vi "Main.vi"() -> ()   [LabVIEW 2020]
uses:
  Global Variables/Global Number of Indices.vi
  Global Variables/Global Correct Answer.vi
  Global Variables/Global N-Back Setting.vi
  Global Variables/Global User_Answer.vi
  Global Variables/Global Label.vi
  Global Variables/Training_Status.vi
  Global Variables/Number_of_Windows.vi
  Global Variables/Window_Size.vi
  Global Variables/Global Send To ANN.vi
  Global Variables/Trainning Done.vi
  Global Variables/Global Difficulty Level.vi
  Global Variables/Global Enable Logging.vi
  Global Variables/Global_Rating.vi
panel:
  out "Difficulty Level":u8
  out "tiggerTime":u32
  out "New square":T1
  out "seq":i8
  out "Data":bool[](array[boolean])
  out "error out":errorcluster
  out "2D Picture":picture
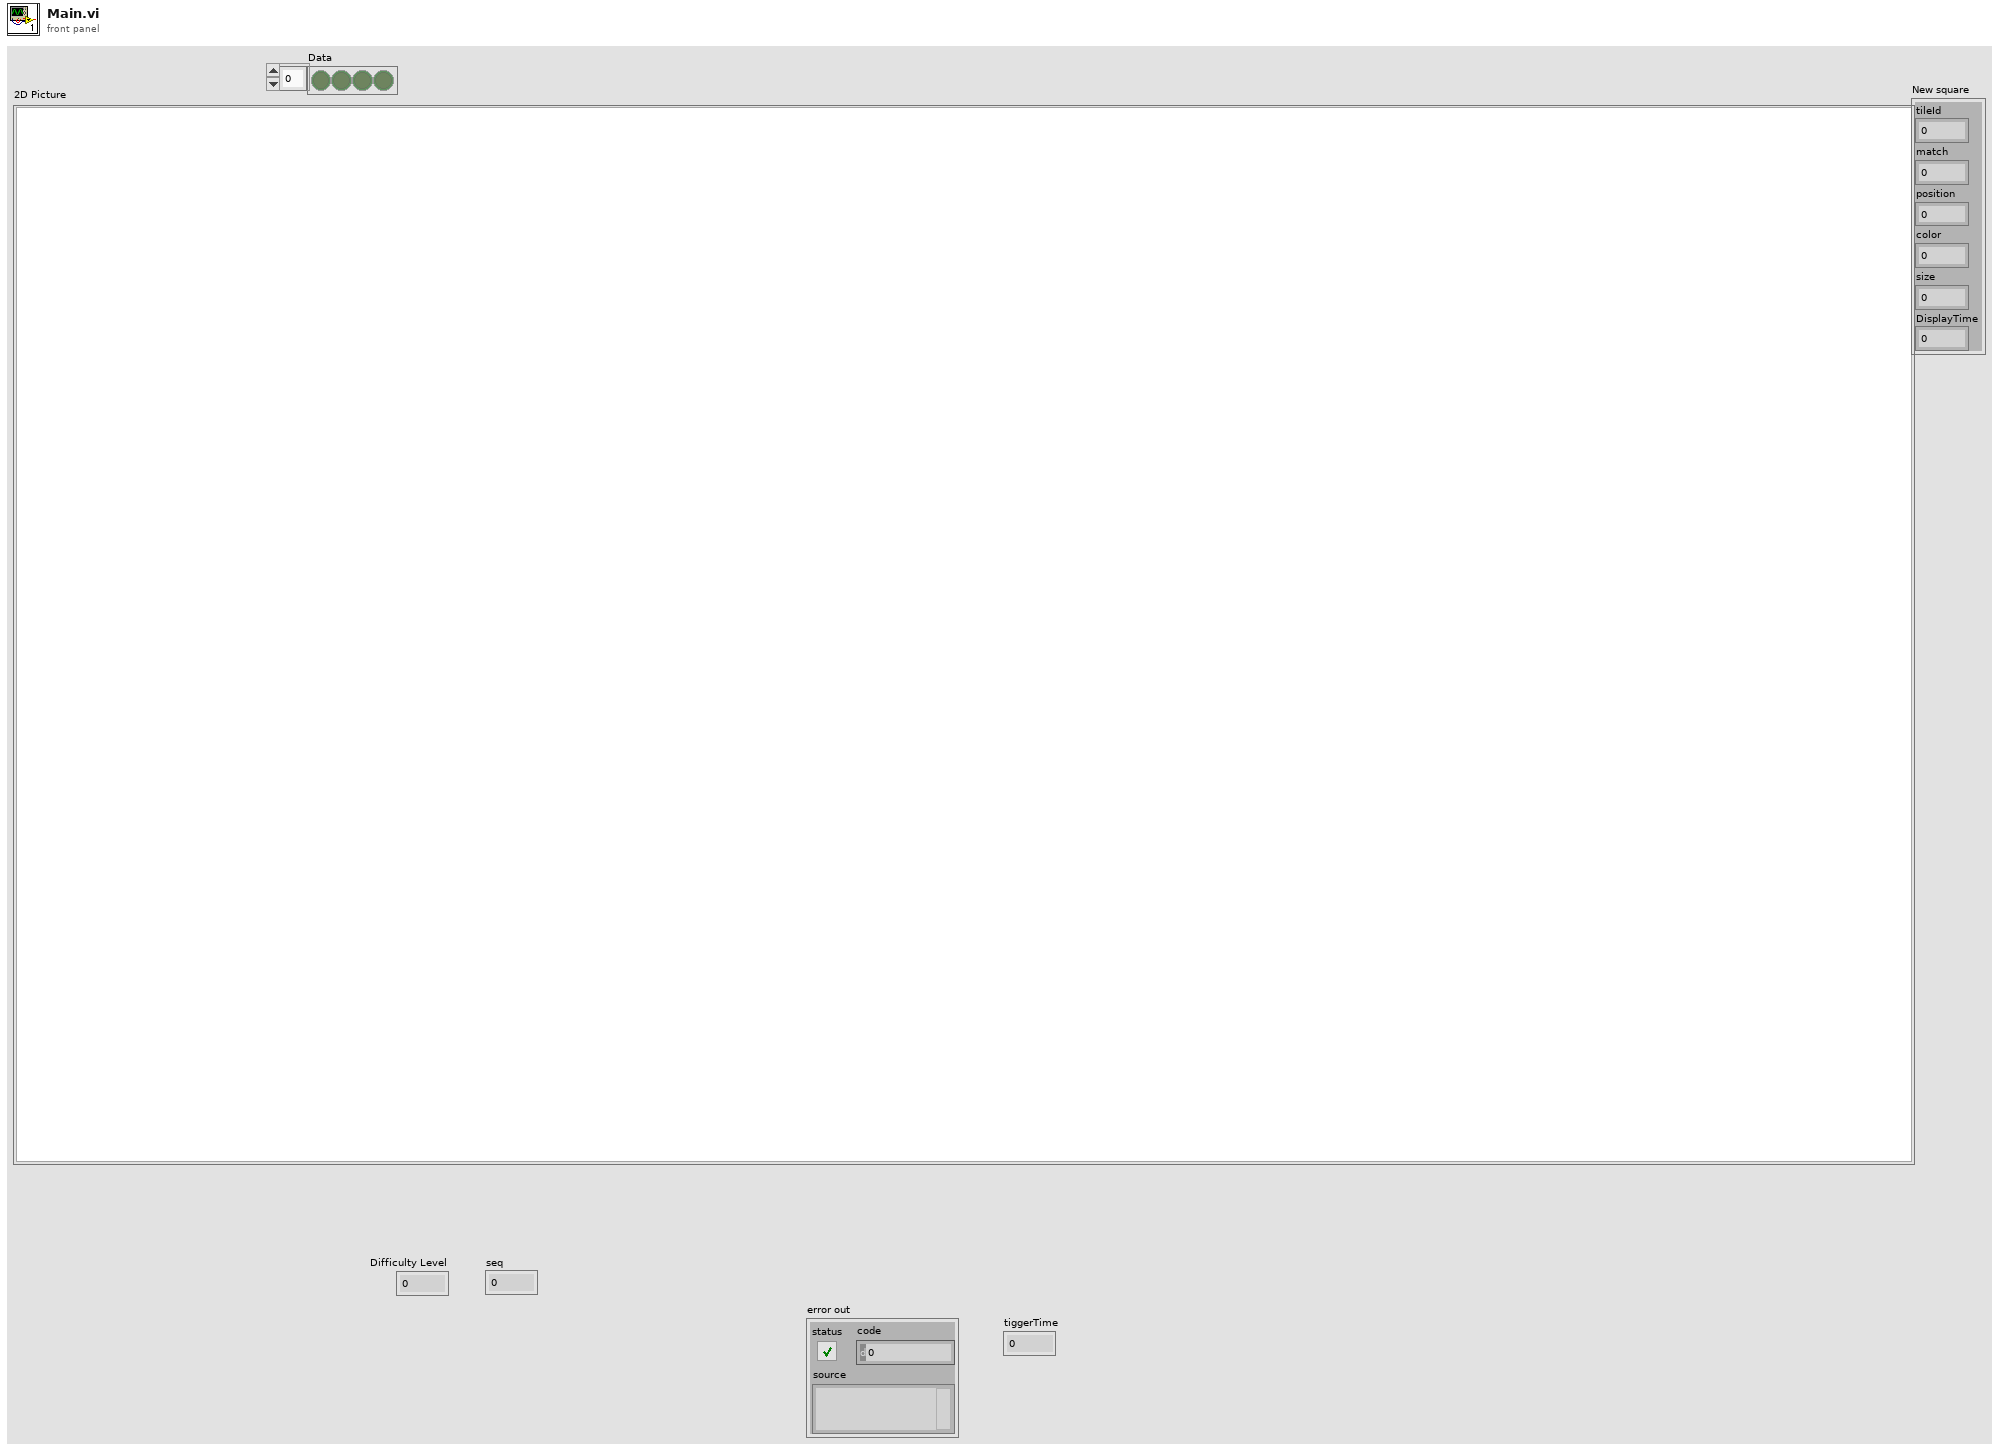
[diagram p1: front panel]
types:
  T1 = cluster{"tileId":i32, "match":i32, "position":i32, "color":u32, "size":i32, "DisplayTime":i32}
  T2 = cluster{"State":i32, "Iteration":i8, "Sequence":i8, "Counter":i8}
  T3 = cluster{"Tile size Y":dbl, "Columns":dbl, "Rows":dbl, "Cross size":dbl, "Offset X":dbl, "Tile size X":dbl, "OffsetY":dbl}
  T4 = cluster{"tileId":i32, "match":i32, "position":i32, "color":u32, "size":i32, "DisplayTime":i32}[]
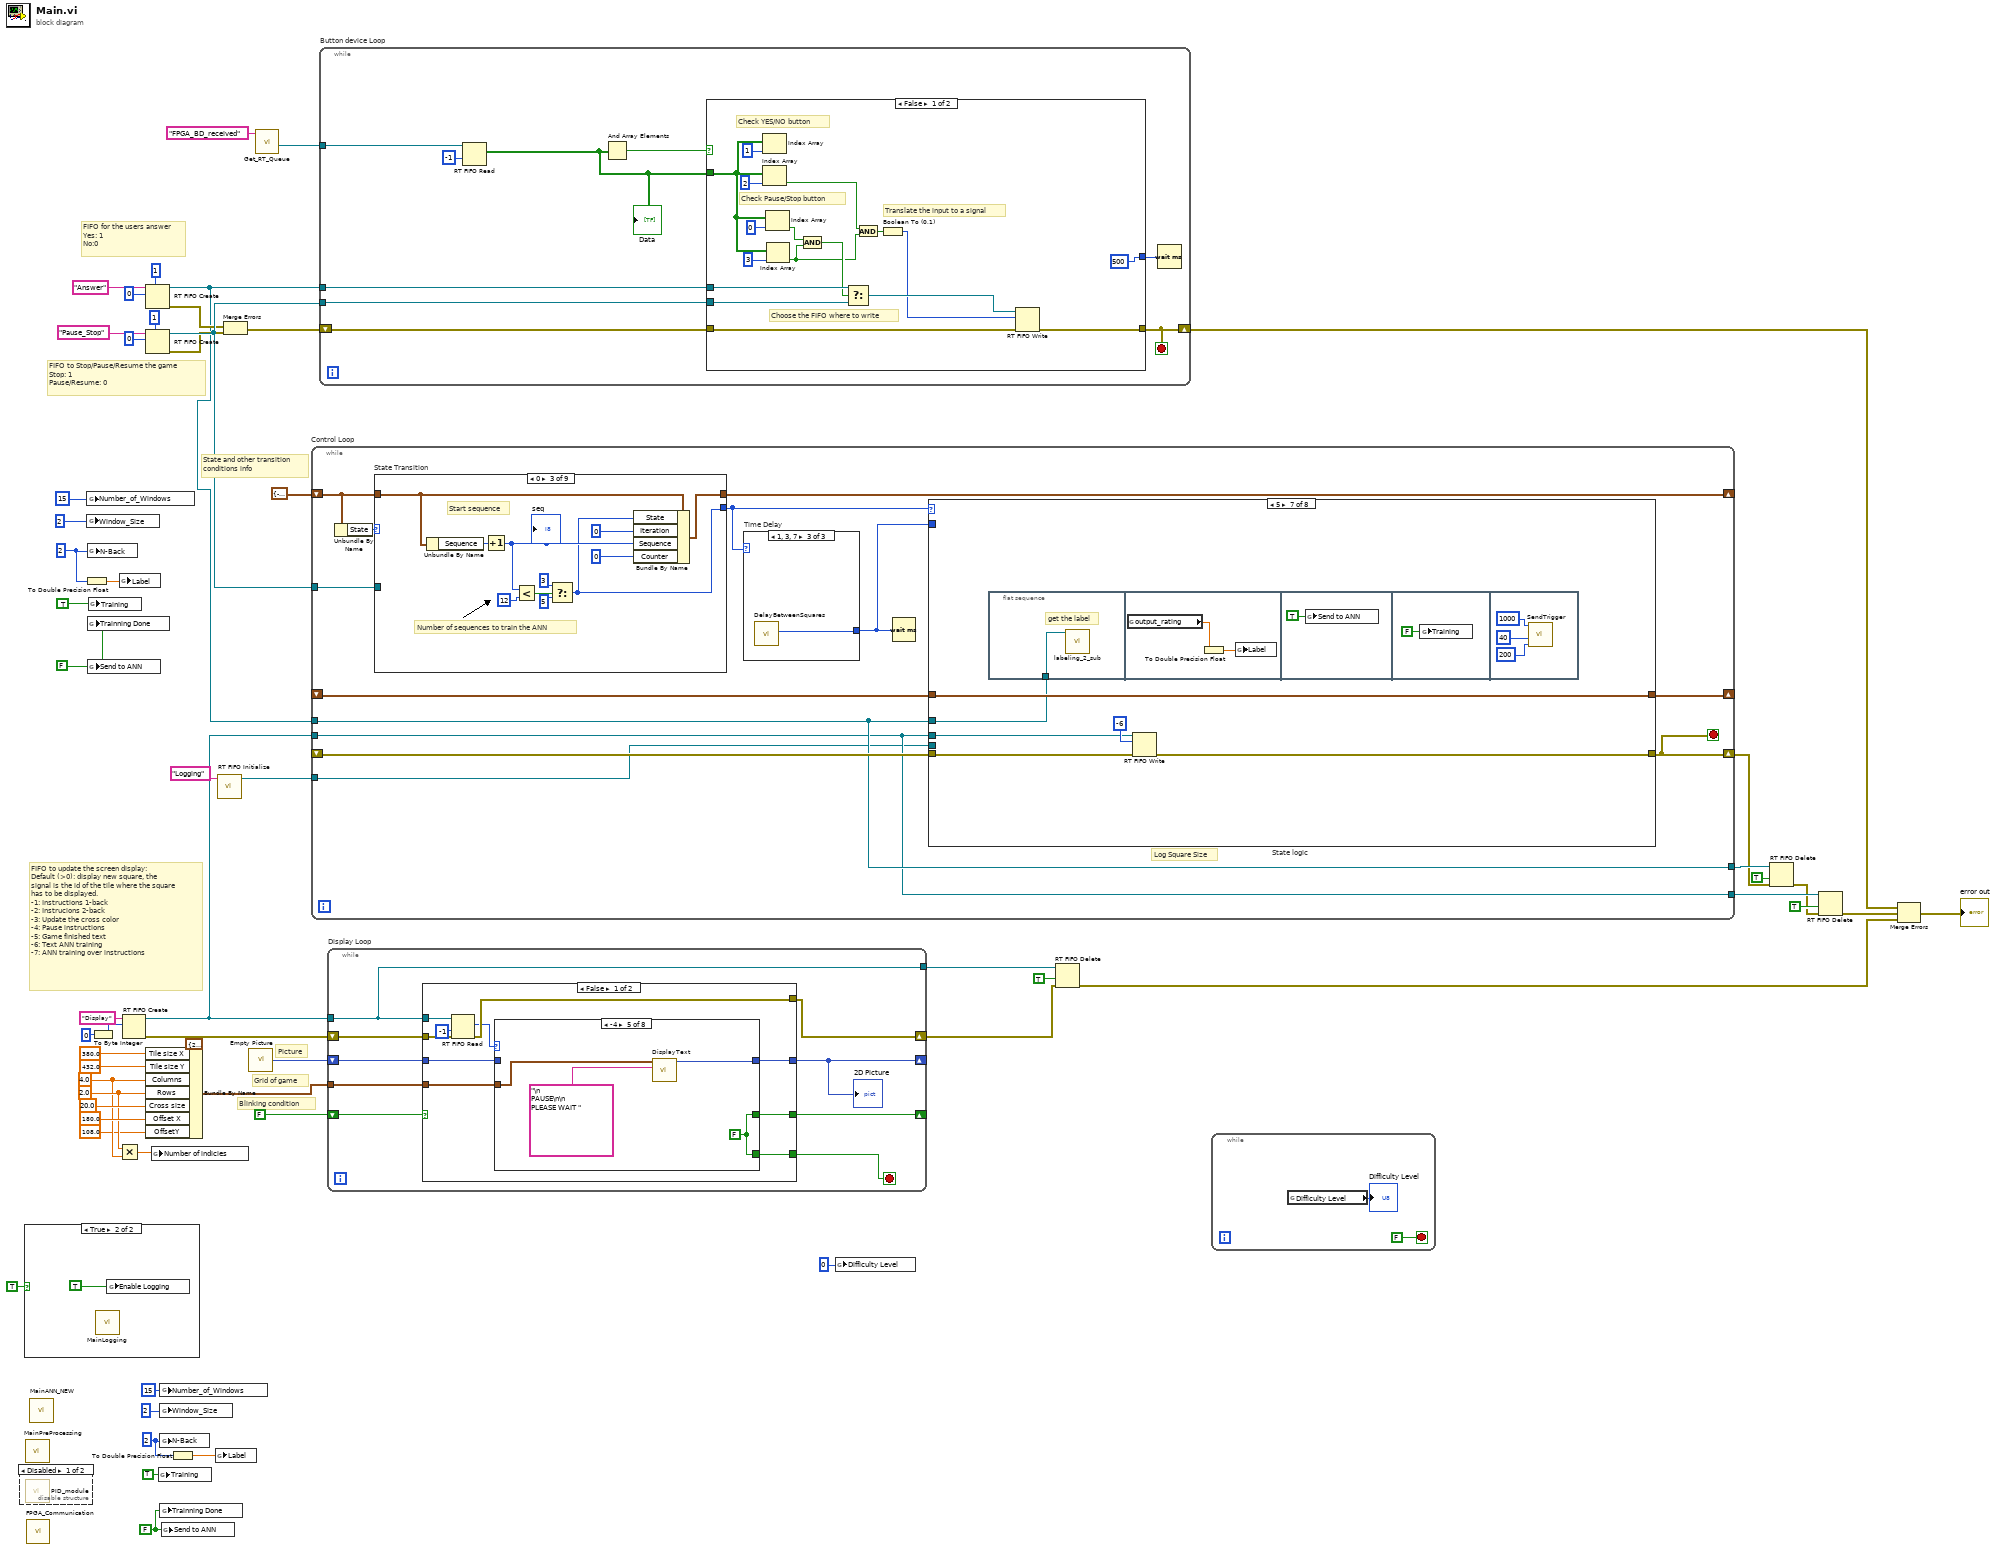
[diagram p0: block diagram]
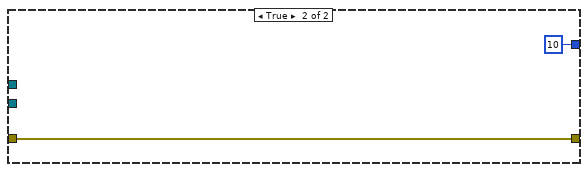
[diagram p3: hidden frame]
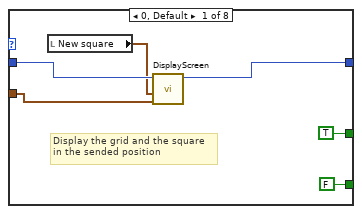
[diagram p5: hidden frame]
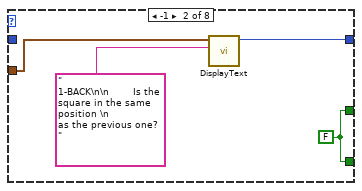
[diagram p6: hidden frame]
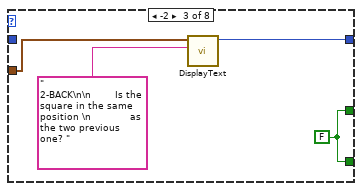
[diagram p7: hidden frame]
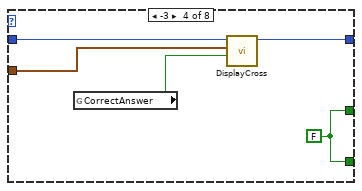
[diagram p8: hidden frame]
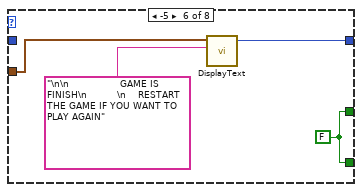
[diagram p9: hidden frame]
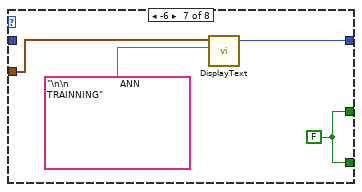
[diagram p10: hidden frame]
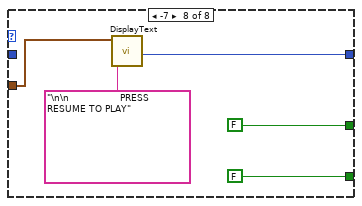
[diagram p11: hidden frame]
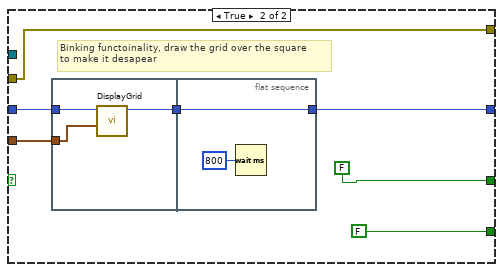
[diagram p12: hidden frame]
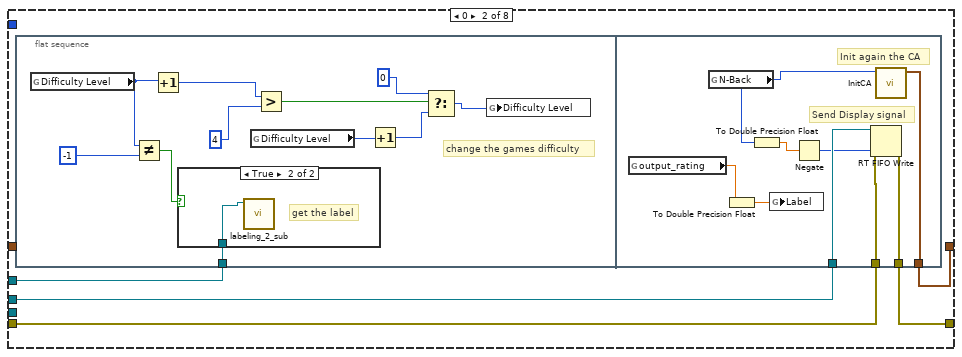
[diagram p14: hidden frame]
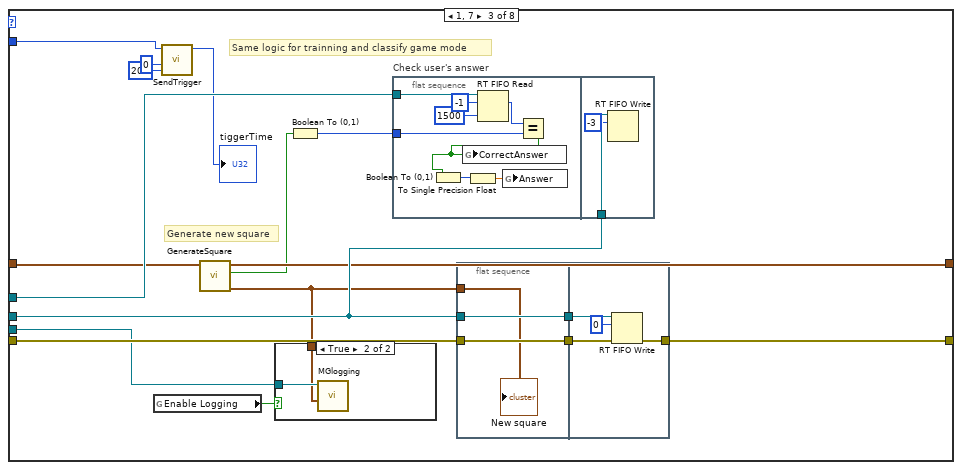
[diagram p16: hidden frame]
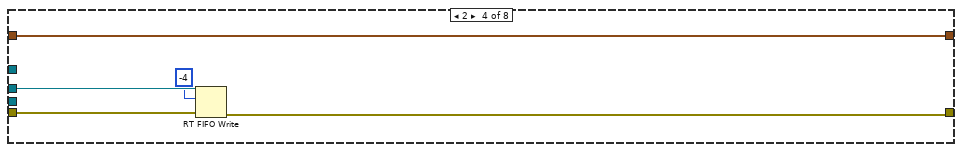
[diagram p18: hidden frame]
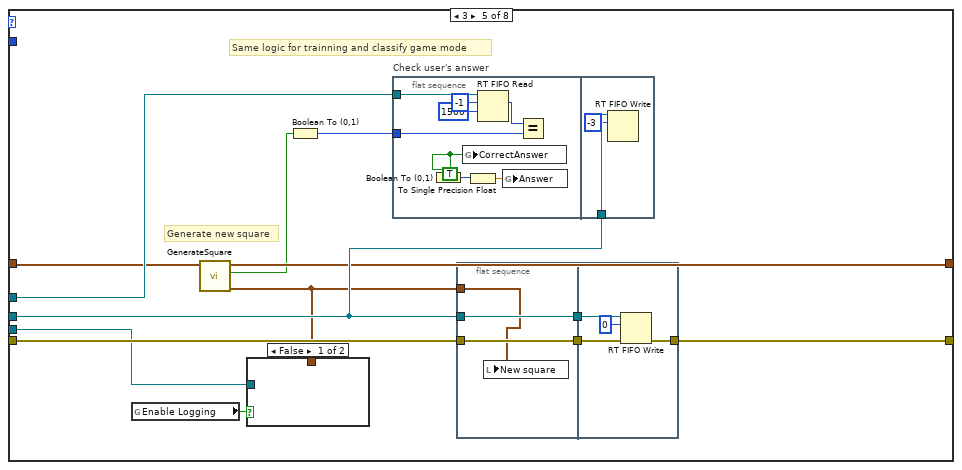
[diagram p19: hidden frame]
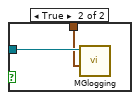
[diagram p20: hidden frame]
diagram:
  w6 = FALSE ("Send to ANN")
  w7 = u8 2 ("N-Back")
  w17 = FALSE ("Send to ANN")
  w18 = u8 2 ("N-Back")
  w47 = 2.0 ("Rows")
  w46 = 4.0 ("Columns")
  # "State and other transition \nconditions info"
  # "Picture"
  # "Grid of game"
  # "Blinking condition"
  # "FIFO to update the screen display:\nDefault (>0): display new square, the \nsignal is the id of the tile where the square\nhas to be displayed.\n-1: Instructions 1-back \n-2: Instrucions 2-back\n-3: Update the cross color \n-4: Pause instructions \n-5: Game finished text\n-6: Text ANN training\n-7: ANN training over instructions"
  # "FIFO to Stop/Pause/Resume the game\nStop: 1\nPause/Resume: 0"
  # "FIFO for the users answer\nYes: 1\nNo:0"
  n1 = disable-structure shown="Disabled" {
    frame Disabled {
      n2 = call "PID_module.vi"() -> ()  [unwired: 11 in]
    }
    frame Enabled {
    }
  }
  n3 = case shown="True" TRUE {
    frame False {
    }
    frame True {
      n4 = call "MainLogging.vi"() -> ()  [unwired: 7 in]
      n5 = global write "Global Enable Logging.vi" "Enable Logging"(TRUE ("Enable Logging")) -> ()
    }
  }
  n6 = call "MainPreProcessing.vi"() -> ()  [unwired: 12 in]
  n7 = call "FPGA_Communication.vi"() -> ()  [unwired: 12 in]
  n8 = call "MainANN_NEW.vi"() -> ()  [unwired: 12 in]
  n9 = To Double Precision Float(number=w18) -> (double precision float=w19:dbl)
  n10 = global write "Number_of_Windows.vi" "Number_of_Windows"(u32 15 ("Number of Windows")) -> ()
  n11 = global write "Window_Size.vi" "Window_Size"(u32 2 ("Window_Size")) -> ()
  n12 = global write "Global N-Back Setting.vi" "N-Back"(w18) -> ()
  n13 = global write "Trainning Done.vi" "Trainning Done"(w17) -> ()
  n14 = global write "Global Send To ANN.vi" "Send to ANN"(w17) -> ()
  n15 = global write "Training_Status.vi" "Training"(TRUE ("Training")) -> ()
  n16 = To Byte Integer(number=0) -> (8bit integer=w57:i8)
  n17 = Multiply(x=w47, y=w46) -> (x*y=w48:dbl)
  n18 = global write "Global Label.vi" "Label"(w19) -> ()
  n19 = RT FIFO Create(0:"Display" ("name (unnamed)"), 1:w57) -> (8:w55:refnum<k33>, 11:w37:errorcluster)  [unwired: 6 in, 1 out]
  n20 = Bundle By Name(cluster=T3 {"Tile size Y"=250.0, "Columns"=4.0, "Rows"=2.0, "Cross size"=20.0, "Offset X"=98.0, "Tile size X"=250.0, "OffsetY"=98.0} ("Grid"), "Tile size X"=380.0, "Tile size Y"=432.0 ("Tile size"), "Columns"=w46, "Rows"=w47, "Cross size"=20.0, "Offset X"=180.0 ("Offset"), "OffsetY"=108.0) -> (w36:T3)
  n21 = RT FIFO Create(0:"Answer" ("name (unnamed)"), 1:i16 0, 4:u32 1 ("size (10)")) -> (8:w1:refnum<k33>, 11:w41:errorcluster)  [unwired: 5 in, 1 out]
  n22 = RT FIFO Create(0:"Pause_Stop" ("name (unnamed)"), 1:i16 0, 4:u32 1 ("size (10)")) -> (8:w45:refnum<k33>, 11:w40:errorcluster)  [unwired: 5 in, 1 out]
  n23 = global write "Global Number of Indices.vi" "Number of indicies"(w48) -> ()
  n24 = global write "Training_Status.vi" "Training"(TRUE ("Training")) -> ()
  n25 = global write "Number_of_Windows.vi" "Number_of_Windows"(u32 15 ("Number of Windows")) -> ()
  n26 = global write "Window_Size.vi" "Window_Size"(u32 2 ("Window_Size")) -> ()
  n27 = global write "Global N-Back Setting.vi" "N-Back"(w7) -> ()
  n28 = global write "Trainning Done.vi" "Trainning Done"(w6) -> ()
  n29 = global write "Global Send To ANN.vi" "Send to ANN"(w6) -> ()
  n30 = To Double Precision Float(number=w7) -> (double precision float=w8:dbl)
  n31 = global write "Global Label.vi" "Label"(w8) -> ()
  n32 = call "RT FIFO Initialize.vi"("name (unnamed)"="Logging") -> ("rt fifo"=w13:refnum<k33>)  [unwired: 9 in, 1 out]
  n33 = Merge Errors(w41, w40) -> (w39:errorcluster)
  n34 = call "Empty Picture"() -> ("empty picture"=w53:picture)
  n35 = call "Get_RT_Queue.vi"("String"="FPGA_BD_received") -> ("rt fifo boolean"=w4:refnum<k33>)  [unwired: 8 in, 2 out]
  n36 = while "Control Loop" {
    tunnel: w55 -> [w64]
    tunnel: w1 -> [w65]
    tunnel: w45 -> [w71]
    shift-right: [w72] -> _
    shift-left: T2 {"State"=-1, "Iteration"=0, "Sequence"=0, "Counter"=0} -> [w73]
    shift-right: [w63] -> _
    shift-left: _ -> [w69]
    shift-right: [w66] -> w32
    shift-left: _ -> [w68]
    tunnel: [w65] -> w34
    tunnel: [w64] -> w33
    tunnel: w13 -> [w62]
    stop <- w66 stop-if-true
    # "Log Square Size"
    n37 = Unbundle By Name(w73) -> ("State"=w74:i32)
    n38 = case "State Transition" shown="0" w74 {
      tunnel: w73 -> [w206 w216 w225 w245 w260 w268 w283 w300 w311]
      tunnel: [w205 w211 w226 w244 w258 w269 w284 w299 w310] -> w72
      tunnel: w71 -> [_ _ _ w243 w256 w267 _ w301 w309]
      tunnel: [w204 0 ("f") w218 w228 w257 w264 w282 w298 w302] -> w70
      frame Default {
        w204 = -4 ("State")
        n39 = Bundle By Name(cluster=w206, "State"=w204, "Iteration"=i8 0, "Sequence"=i8 0, "Counter"=i8 0) -> (w205:T2)
      }
      frame -1 {
        # "Start state"
        n40 = Bundle By Name(cluster=w216, "State"=0, "Iteration"=i8 -1, "Sequence"=i8 0, "Counter"=i8 0) -> (w211:T2)
      }
      frame 0 {
        # "Start sequence"
        # "Number of sequences to train the ANN"
        n41 = Unbundle By Name(w225) -> ("Sequence"=w224:i8)
        n42 = Increment(x=w224) -> (x+1=w220:i8)
        "seq" <- w220
        n43 = Less?(x=w220, y=12) -> (x < y?=w223:bool)
        n44 = Select(t=3 ("State"), s=w223, f=5) -> (s? t:f=w218:i32)
        n45 = Bundle By Name(cluster=w225, "State"=w218, "Iteration"=i8 0 ("Sequence"), "Sequence"=w220, "Counter"=i8 0) -> (w226:T2)
      }
      frame 1 {
        # "Check for Pause signal"
        # "Increase iteration number"
        # "Playing in trainning mode"
        n46 = Unbundle By Name(w245) -> ("Iteration"=w250:i8, "Sequence"=w235:i8)
        n47 = RT FIFO Read(0:w243, 1:i8 -1 ("element")) -> (9:w241:i16)  [unwired: 2 in, 4 out]
        n48 = Increment(x=w250) -> (x+1=w248:i8)
        n49 = Equal?(x=w241, y=i8 0) -> (x = y?=w238:bool)
        n50 = Less?(x=w248, y=i8 7) -> (x < y?=w237:bool)
        n51 = Select(t=1 ("State"), s=w237, f=0) -> (s? t:f=w236:i32)
        n52 = Equal?(x=w235, y=i8 2) -> (x = y?=w232:bool)
        n53 = Select(t=2, s=w238, f=w236) -> (s? t:f=w229:i32)
        n54 = Equal To 0?(x=w236) -> (x = 0?=w233:bool)
        n55 = And(x=w232, y=w233) -> (x .and. y?=w231:bool)
        n56 = Select(t=5, s=w231, f=w229) -> (s? t:f=w228:i32)
        n57 = Bundle By Name(cluster=w245, "State"=w228, "Iteration"=w248, "Sequence"=w235, "Counter"=i8 0) -> (w244:T2)
      }
      frame 2 {
        # "Waits untill it gets a Stop/Pause signal"
        # "Pause State"
        n58 = global read "Trainning Done.vi" "Trainning Done"() -> (w255:bool)
        n59 = RT FIFO Read(0:w256, 2:-1 ("timeout in ms (0)")) -> (9:w262:i16)  [unwired: 2 in, 4 out]
        n60 = Equal To 0?(x=w262) -> (x = 0?=w261:bool)
        n61 = Select(t=7, s=w255, f=3 ("timeout in ms (0)")) -> (s? t:f=w252:i32)
        n62 = Select(t=w252, s=w261, f=4) -> (s? t:f=w257:i32)
        n63 = Bundle By Name(cluster=w260, "State"=w257) -> (w258:T2)
      }
      frame 3 {
        # "State: back to normal"
        n64 = Unbundle By Name(w268) -> ("Sequence"=w276:i8, "Counter"=w266:i8)
        n65 = RT FIFO Read(0:w267, 1:i8 -1 ("element")) -> (9:w274:i16)  [unwired: 2 in, 4 out]
        n66 = Increment(x=w266) -> (x+1=w265:i8)
        n67 = Equal?(x=w274, y=i8 1) -> (x = y?=w272:bool)
        n68 = Less?(x=w265, y=i8 3) -> (x < y?=w279:bool)
        n69 = Select(t=3 ("State"), s=w279, f=1) -> (s? t:f=w271:i32)
        n70 = Select(t=2, s=w272, f=w271) -> (s? t:f=w264:i32)
        n71 = Bundle By Name(cluster=w268, "State"=w264, "Sequence"=w276, "Counter"=w265) -> (w269:T2)
      }
      frame 5 {
        # "State to wait untill the ANN is trained"
        n72 = while {
          tunnel: [w287] -> w284
          tunnel: w283 -> [w286]
          tunnel: [w285] -> w282
          stop <- w291 stop-if-true
          w285 = 6 ("State")
          n73 = global read "Trainning Done.vi" "Trainning Done"() -> (w291:bool)
          n74 = Bundle By Name(cluster=w286, "State"=w285, "Iteration"=i8 0, "Sequence"=i8 0, "Counter"=i8 0) -> (w287:T2)
        }
        n75 = Wait (ms)(milliseconds to wait=u32 1500) -> ()  [unwired: 1 out]
      }
      frame 6 {
        w298 = 7 ("s? t:f")
        # "State to wait to start to play classify"
        n76 = RT FIFO Read(0:w301, 2:-1 ("timeout in ms (0)")) -> (9:w296:i16)  [unwired: 2 in, 4 out]
        n77 = global write "Global Difficulty Level.vi" "Difficulty Level"(u8 1 ("Difficulty Level")) -> ()
        n78 = Equal To 0?(x=w296) -> (x = 0?=w295:bool)
        n79 = Select(t=7 ("timeout in ms (0)"), s=w295, f=4) -> ()  [unwired: 1 out]
        n80 = Bundle By Name(cluster=w300, "State"=w298) -> (w299:T2)
      }
      frame 7 {
        # "Check for pause signal"
        # "Playing classification"
        n81 = RT FIFO Read(0:w309, 1:i8 -1 ("element")) -> (9:w307:i16)  [unwired: 2 in, 4 out]
        n82 = Equal?(x=w307, y=i8 0) -> (x = y?=w305:bool)
        n83 = Select(t=2, s=w305, f=7) -> (s? t:f=w302:i32)
        n84 = Bundle By Name(cluster=w311, "State"=w302, "Counter"=i8 0) -> (w310:T2)
      }
    }
    n85 = case "Time Delay" shown="1, 3, 7" w70 {
      tunnel: [0 ("f") i64 6000 ("f") w203] -> w67
      frame Default {
      }
      frame 0 {
        # "The instructions/Text\nis displaed for 4 s"
      }
      frame 1, 3, 7 {
        n86 = call "DelayBetweenSquares.vi"() -> ("milliseconds to wait"=w203:u32)  [unwired: 10 in]
      }
    }
    n87 = Wait (ms)(milliseconds to wait=w67) -> ()  [unwired: 1 out]
    n88 = case "State logic" shown="5" w70 {
      tunnel: w64 -> [_ w80 w115 w143 w152 w179 w185 w198]
      tunnel: w65 -> [_ w77 w117 _ w154 _ w181 _]
      tunnel: w69 -> [w75 _ w113 w139 w150 w176 w182 _]
      tunnel: w68 -> [w76 w79 w118 w142 w155 w178 w184 w199]
      tunnel: [w76 w78 w119 w141 w156 w177 w183 w197] -> w66
      tunnel: w67 -> [_ _ w109 _ _ _ _ _]
      tunnel: [w75 w81 w114 w139 w151 w176 w182 w195] -> w63
      tunnel: w62 -> [_ _ w106 _ w146 _ _ _]
      frame Default {
      }
      frame 0 {
        n89 = flat-sequence {
          tunnel: w77 -> [w82]
          tunnel: [w101] -> w81
          tunnel: w80 -> [w99]
          tunnel: w79 -> [w97]
          tunnel: [w96] -> w78
          frame #0 {
            # "change the games difficulty"
            n90 = global read "Global Difficulty Level.vi" "Difficulty Level"() -> (w85:u8)
            n91 = Not Equal?(x=w85, y=-1) -> (x != y?=w83:bool)
            n92 = Increment(x=w85) -> (x+1=w92:u8)
            n93 = case shown="True" w83 {
              tunnel: w82 -> [_ w93]
              frame False {
              }
              frame True {
                # "get the label"
                n94 = call "labeling_2_sub.vi"("Refnum in"=w93) -> ()  [unwired: 9 in, 2 out]
              }
            }
            n95 = global read "Global Difficulty Level.vi" "Difficulty Level"() -> (w90:u8)
            n96 = Greater?(x=w92, y=4) -> (0:w87:bool)
            n97 = Increment(x=w90) -> (x+1=w89:u8)
            n98 = Select(t=0, s=w87, f=w89) -> (s? t:f=w86:i32)
            n99 = global write "Global Difficulty Level.vi" "Difficulty Level"(w86) -> ()
          }
          frame #1 {
            # "Send Display signal"
            # "Init again the CA"
            n100 = global read "Global_Rating.vi" "output_rating"() -> (w95:dbl)
            n101 = global read "Global N-Back Setting.vi" "N-Back"() -> (w102:u8)
            n102 = To Double Precision Float(number=w95) -> (double precision float=w94:dbl)
            n103 = To Double Precision Float(number=w102) -> (double precision float=w100:dbl)
            n104 = global write "Global Label.vi" "Label"(w94) -> ()
            n105 = Negate(x=w100) -> (-x=w98:i8)
            n106 = RT FIFO Write(0:w99, 1:w98, 3:w97) -> (11:w96:errorcluster)  [unwired: 2 in, 3 out]
            n107 = call "InitCA.vi"("N-Back"=w102) -> ("CA"=w101:T4)  [unwired: 10 in]
          }
        }
      }
      frame 1, 7 {
        # "Same logic for trainning and classify game mode"
        # "Generate new square"
        n108 = global read "Global Enable Logging.vi" "Enable Logging"() -> (w104:bool)
        n109 = call "SendTrigger.vi"("System Exe time"=200, "Window time"=0, "TimeSquares"=w109) -> ("millisecond timer value"=→"tiggerTime":u32)  [unwired: 8 in]
        n110 = call "GenerateSquare.vi"("CA"=w113) -> ("New square"=w105:T1, "Match"=w110:bool, "updated CA"=w114:T4)  [unwired: 8 in]
        n111 = case shown="True" w104 {
          tunnel: w106 -> [_ w121]
          tunnel: w105 -> [_ w120]
          frame False {
          }
          frame True {
            n112 = call "MGlogging.vi"("New square"=w120, "Refnum in"=w121) -> ()  [unwired: 9 in, 1 out]
          }
        }
        n113 = Boolean To (0,1)(Boolean=w110) -> (0, 1=w116:i16)
        n114 = flat-sequence "Check user's answer" {
          tunnel: w117 -> [w136]
          tunnel: w116 -> [w132]
          tunnel: w115 -> [w138]
          frame #0 {
            n115 = RT FIFO Read(0:w136, 1:i16 -1 ("element"), 2:1500 ("timeout in ms (0)")) -> (9:w133:i16)  [unwired: 1 in, 4 out]
            n116 = Equal?(x=w133, y=w132) -> (x = y?=w129:bool)
            n117 = Boolean To (0,1)(Boolean=w129) -> (0, 1=w131:i16)
            n118 = global write "Global Correct Answer.vi" "CorrectAnswer"(w129) -> ()
            n119 = To Single Precision Float(number=w131) -> (single precision float=w130:sgl)
            n120 = global write "Global User_Answer.vi" "Answer"(w130) -> ()
          }
          frame #1 {
            n121 = RT FIFO Write(0:w138, 1:i8 -3 ("element")) -> ()  [unwired: 3 in, 4 out]
          }
        }
        n122 = flat-sequence {
          tunnel: w115 -> [w123]
          tunnel: w118 -> [w124]
          tunnel: [w124] -> w112
          tunnel: [w123] -> w111
          tunnel: w105 -> [w122]
          tunnel: [w128] -> w119
          tunnel: w112 -> [w127]
          tunnel: w111 -> [w126]
          frame #0 {
            "New square" <- w122
          }
          frame #1 {
            n123 = RT FIFO Write(0:w126, 1:i8 0 ("element"), 3:w127) -> (11:w128:errorcluster)  [unwired: 2 in, 3 out]
          }
        }
      }
      frame 2 {
        n124 = RT FIFO Write(0:w143, 1:i8 -4 ("element"), 3:w142) -> (11:w141:errorcluster)  [unwired: 2 in, 3 out]
      }
      frame 3 {
        # "Same logic for trainning and classify game mode"
        # "Generate new square"
        n125 = global read "Global Enable Logging.vi" "Enable Logging"() -> (w144:bool)
        n126 = call "GenerateSquare.vi"("CA"=w150) -> ("New square"=w145:T1, "Match"=w147:bool, "updated CA"=w151:T4)  [unwired: 8 in]
        n127 = case shown="False" w144 {
          tunnel: w146 -> [_ w158]
          tunnel: w145 -> [_ w157]
          frame False {
          }
          frame True {
            n128 = call "MGlogging.vi"("New square"=w157, "Refnum in"=w158) -> ()  [unwired: 9 in, 1 out]
          }
        }
        n129 = Boolean To (0,1)(Boolean=w147) -> (0, 1=w153:i16)
        n130 = flat-sequence "Check user's answer" {
          tunnel: w154 -> [w173]
          tunnel: w153 -> [w169]
          tunnel: w152 -> [w175]
          frame #0 {
            w166 = TRUE ("CorrectAnswer")
            n131 = Boolean To (0,1)(Boolean=w166) -> (0, 1=w168:i16)
            n132 = global write "Global Correct Answer.vi" "CorrectAnswer"(w166) -> ()
            n133 = To Single Precision Float(number=w168) -> (single precision float=w167:sgl)
            n134 = RT FIFO Read(0:w173, 1:i16 -1 ("element"), 2:1500 ("timeout in ms (0)")) -> (9:w170:i16)  [unwired: 1 in, 4 out]
            n135 = global write "Global User_Answer.vi" "Answer"(w167) -> ()
            n136 = Equal?(x=w170, y=w169) -> ()  [unwired: 1 out]
          }
          frame #1 {
            n137 = RT FIFO Write(0:w175, 1:i8 -3 ("element")) -> ()  [unwired: 3 in, 4 out]
          }
        }
        n138 = flat-sequence {
          tunnel: w152 -> [w160]
          tunnel: w155 -> [w161]
          tunnel: [w161] -> w149
          tunnel: [w160] -> w148
          tunnel: w145 -> [w159]
          tunnel: [w165] -> w156
          tunnel: w149 -> [w164]
          tunnel: w148 -> [w163]
          frame #0 {
            n139 = local write "New square"(w159) -> ()
          }
          frame #1 {
            n140 = RT FIFO Write(0:w163, 1:i8 0 ("element"), 3:w164) -> (11:w165:errorcluster)  [unwired: 2 in, 3 out]
          }
        }
      }
      frame 4 {
        n141 = RT FIFO Write(0:w179, 1:i8 -5 ("element"), 3:w178) -> (11:w177:errorcluster)  [unwired: 2 in, 3 out]
      }
      frame 5 {
        n142 = flat-sequence {
          tunnel: w181 -> [w187]
          frame #0 {
            # "get the label"
            n143 = call "labeling_2_sub.vi"("Refnum in"=w187) -> ()  [unwired: 9 in, 2 out]
          }
          frame #1 {
            n144 = global read "Global_Rating.vi" "output_rating"() -> (w189:dbl)
            n145 = To Double Precision Float(number=w189) -> (double precision float=w188:dbl)
            n146 = global write "Global Label.vi" "Label"(w188) -> ()
          }
          frame #2 {
            n147 = global write "Global Send To ANN.vi" "Send to ANN"(TRUE ("Send to ANN")) -> ()
          }
          frame #3 {
            n148 = global write "Training_Status.vi" "Training"(FALSE ("Training")) -> ()
          }
          frame #4 {
            n149 = call "SendTrigger.vi"("System Exe time"=200, "Window time"=40, "TimeSquares"=1000) -> ()  [unwired: 8 in, 1 out]
          }
        }
        n150 = RT FIFO Write(0:w185, 1:i8 -6 ("element"), 3:w184) -> (11:w183:errorcluster)  [unwired: 2 in, 3 out]
      }
      frame 6 {
        # "Init the CA for the classify mode"
        n151 = global read "Global N-Back Setting.vi" "N-Back"() -> (w196:u8)
        n152 = RT FIFO Write(0:w198, 1:i8 -7 ("element"), 3:w199) -> (11:w197:errorcluster)  [unwired: 2 in, 3 out]
        n153 = call "InitCA.vi"("N-Back"=w196) -> ("CA"=w195:T4)  [unwired: 10 in]
      }
    }
  }
  n154 = while "Button device Loop" {
    tunnel: w1 -> [w321]
    tunnel: w45 -> [w320]
    shift-right: [w318] -> w28
    shift-left: w39 -> [w319]
    tunnel: w4 -> [w316]
    stop <- w318 stop-if-true
    n155 = RT FIFO Read(0:w316, 2:-1 ("timeout in ms (0)")) -> (9:w314:bool[])  [unwired: 2 in, 4 out]
    "Data" <- w314
    n156 = And Array Elements(Boolean array=w314) -> (logical AND=w317:bool)
    n157 = case shown="False" w317 {
      tunnel: w314 -> [w332 _]
      tunnel: w321 -> [w338 _]
      tunnel: w320 -> [w337 _]
      tunnel: w319 -> [w326 w340]
      tunnel: [w325 w340] -> w318
      tunnel: [500 ("index") 10 ("index")] -> w313
      frame False {
        # "Translate the input to a signal"
        # "Choose the FIFO where to write"
        # "Check Pause/Stop button"
        # "Check YES/NO button"
        n158 = Index Array(array=w332, index=1) -> ()  [unwired: 1 out]
        n159 = Index Array(array=w332, index=2) -> (element=w330:bool)
        n160 = Index Array(array=w332, index=0) -> (element=w324:bool)
        n161 = Index Array(array=w332, index=3) -> (element=w323:bool)
        n162 = And(x=w324, y=w323) -> (x .and. y?=w331:bool)
        n163 = Select(t=w338, s=w331, f=w337) -> (s? t:f=w328:refnum<k33>)
        n164 = And(x=w330, y=w323) -> (x .and. y?=w329:bool)
        n165 = Boolean To (0,1)(Boolean=w329) -> (0, 1=w327:i16)
        n166 = RT FIFO Write(0:w328, 1:w327, 3:w326) -> (11:w325:errorcluster)  [unwired: 2 in, 3 out]
      }
      frame True {
      }
    }
    n167 = Wait (ms)(milliseconds to wait=w313) -> ()  [unwired: 1 out]
  }
  n168 = while "Display Loop" {
    tunnel: w55 -> [w343]
    shift-right: [w348] -> _
    shift-left: FALSE -> [w349]
    shift-right: [w346] -> _
    shift-left: w53 -> [w347]
    tunnel: w36 -> [w345]
    tunnel: [w343] -> w38
    shift-right: [w341] -> w16
    shift-left: w37 -> [w342]
    stop <- w344 stop-if-true
    n169 = case shown="False" w349 {
      tunnel: [w354 FALSE] -> w348
      tunnel: w347 -> [w357 w400]
      tunnel: [w355 w399] -> w346
      tunnel: w345 -> [w356 w398]
      tunnel: w343 -> [w359 _]
      tunnel: [w353 FALSE] -> w344
      tunnel: w342 -> [w352 w396]
      tunnel: [w351 w396] -> w341
      frame False {
        n170 = RT FIFO Read(0:w359, 2:-1 ("timeout in ms (0)"), 3:w352) -> (9:w350:i8, 11:w351:errorcluster)  [unwired: 1 in, 3 out]
        n171 = case shown="-4" w350 {
          tunnel: [TRUE w367 w371 w374 w379 w383 w387 FALSE] -> w354
          tunnel: [w362 w369 w370 w376 w380 w384 w388 w393] -> w355
          tunnel: w357 -> [w364 _ _ w377 _ _ _ _]
          tunnel: w356 -> [w361 w366 w373 w375 w381 w385 w389 w394]
          tunnel: [FALSE w367 w371 w374 w379 w383 w387 FALSE] -> w353
          frame 0, Default {
            # "Display the grid and the square\nin the sended position"
            n172 = local read "New square"() -> (w360:T1)
            n173 = call "DisplayScreen.vi"("Grid"=w361, "square"=w360, "input picture"=w364) -> ("2D Picture"=w362:picture)  [unwired: 8 in]
          }
          frame -1 {
            w367 = FALSE
            n174 = call "DisplayText.vi"("text"="                      1-BACK\n\n        Is the square in the same position \n                as the previous one? ", "Grid"=w366) -> ("new picture"=w369:picture)  [unwired: 9 in]
          }
          frame -2 {
            w371 = FALSE
            n175 = call "DisplayText.vi"("text"="                      2-BACK\n\n        Is the square in the same position \n             as the two previous one? ", "Grid"=w373) -> ("new picture"=w370:picture)  [unwired: 9 in]
          }
          frame -3 {
            w374 = FALSE
            n176 = global read "Global Correct Answer.vi" "CorrectAnswer"() -> (w378:bool)
            n177 = call "DisplayCross.vi"("CorrectAnswer"=w378, "Grid"=w375, "new picture in"=w377) -> ("new picture out"=w376:picture)  [unwired: 8 in]
          }
          frame -4 {
            w379 = FALSE
            n178 = call "DisplayText.vi"("text"="\n                              PAUSE\n\n                   PLEASE WAIT ", "Grid"=w381) -> ("new picture"=w380:picture)  [unwired: 9 in]
          }
          frame -5 {
            w383 = FALSE
            n179 = call "DisplayText.vi"("text"="\n\n                 GAME IS FINISH\n          \n    RESTART THE GAME IF YOU WANT TO PLAY AGAIN", "Grid"=w385) -> ("new picture"=w384:picture)  [unwired: 9 in]
          }
          frame -6 {
            w387 = FALSE
            n180 = call "DisplayText.vi"("text"="\n\n                 ANN TRAINNING", "Grid"=w389) -> ("new picture"=w388:picture)  [unwired: 9 in]
          }
          frame -7 {
            n181 = call "DisplayText.vi"("text"="\n\n                 PRESS RESUME TO PLAY", "Grid"=w394) -> ("new picture"=w393:picture)  [unwired: 9 in]
          }
        }
      }
      frame True {
        # "Binking functoinality, draw the grid over the square\nto make it desapear"
        n182 = flat-sequence {
          tunnel: [w405] -> w401
          tunnel: w400 -> [w404]
          tunnel: w398 -> [w403]
          tunnel: [w406] -> w399
          tunnel: w401 -> [w406]
          frame #0 {
            n183 = call "DisplayGrid.vi"("Grid"=w403, "input picture"=w404) -> ("new picture"=w405:picture)  [unwired: 9 in]
          }
          frame #1 {
            n184 = Wait (ms)(milliseconds to wait=u32 800) -> ()  [unwired: 1 out]
          }
        }
      }
    }
    "2D Picture" <- w346
  }
  n185 = global write "Global Difficulty Level.vi" "Difficulty Level"(u8 0 ("Difficulty Level")) -> ()
  n186 = RT FIFO Delete(0:w38, 2:TRUE ("force destroy? (F)"), 3:w16) -> (11:w26:errorcluster)
  n187 = while {
    stop <- FALSE stop-if-true
    n188 = global read "Global Difficulty Level.vi" "Difficulty Level"() -> (→"Difficulty Level":u8)
  }
  n189 = RT FIFO Delete(0:w34, 2:TRUE ("force destroy? (F)"), 3:w32) -> (11:w29:errorcluster)
  n190 = RT FIFO Delete(0:w33, 2:TRUE ("force destroy? (F)"), 3:w29) -> (11:w27:errorcluster)
  n191 = Merge Errors(w28, w27, w26) -> (→"error out":errorcluster)
